vi "Fetch Repo Details.vi"(8 "error in (no error)":errorcluster) -> (0 "error out":errorcluster, 3 "Repo":refnum<class "Repo.lvclass">)   [LabVIEW 2020, in "Packages.lvlib" / "GPM.lvlib"]
uses:
  GPM.lvlib
  Repo_class/Repo.lvclass
  Repo_class/RepoType--enum.ctl
  Repo_class/Repo.lvclass/Repo.ctl
  Repo_class/Write Name.vi
  Repo_class/Write RepoType.vi
  Repo_class/Write URL.vi
  Repo_class/Write LastUpdated.vi
  <vilib>/addons/database/Connection.llb/DB Tools Open Connec (String).vi
  <vilib>/addons/database/_DB Variant To Data/Database Variant To Data.xnode
  <vilib>/addons/database/NI_Database_API.lvlib
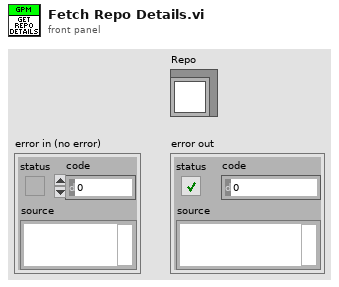
[diagram p1: front panel]
types:
  T1 = typedef "Packages.lvlib/Repo.lvclass/RepoType--enum.ctl" = enum16{"VIPM", "NIPM", "GPM"}
  T2 = typedef "NI_Database_API.lvlib/Conn ObjectReference.ctl" = refnum<k1>
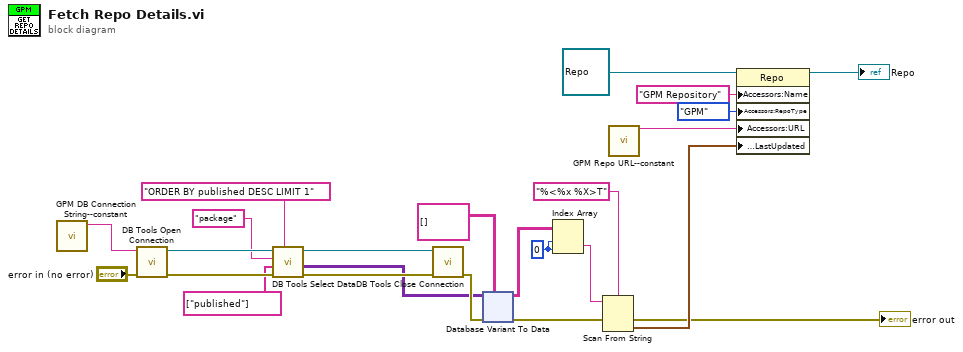
[diagram p0: block diagram]
diagram:
  w12 = 0 ("disabled index (col)")
  n1 = call "GPM DB Connection String--constant.vi"() -> ("DB Connection String"=w5:string)  [unwired: 11 in]
  n2 = call-poly <vilib>:"DB Tools Open Connection.vi"("error in (no error)"="error in (no error)", "connection information"=w5) -> ("error out"=w24:errorcluster, "connection reference"=w14:T2)  [unwired: 6 in]
  n3 = call <vilib>:"DB Tools Select Data.vi"("condition"="ORDER BY published DESC LIMIT 1", "error in (no error)"=w24, "columns"=string[] ["published"], "table"="package", "connection reference"=w14) -> ("error out"=w22:errorcluster, "data"=w20:variant[][], "connection reference out"=w23:T2)  [unwired: 1 in]
  n4 = call <vilib>:"DB Tools Close Connection.vi"("error in (no error)"=w22, "connection reference"=w23) -> ("error out"=w21:errorcluster)  [unwired: 5 in]
  n5 = xnode "Database Variant To Data"("database variant"=w20, "error in (no error)"=w21, "type"=string[][] []) -> ("data"=w17:string[][], "error out"=w11:errorcluster)
  n6 = Index Array(array=w17, index (row)=w12, index (col)=w12) -> (element=w10:string)
  n7 = Scan From String(format string="%<%x %X>T", input string=w10, error in=w11) -> (error out=→"error out":errorcluster, output 1=w3:timestamp)  [unwired: 2 in, 2 out]
  n8 = call "GPM Repo URL--constant.vi"() -> ("GPM Repo URL"=w4:string)  [unwired: 11 in]
  n9 = property class="Repo"(reference=refnum<class "Repo.lvclass"> refnum ("Repo in"), "Accessors:Name"="GPM Repository" ("Name"), "Accessors:RepoType"=RepoType--enum."GPM" ("RepoType"), "Accessors:URL"=w4, "Accessors:LastUpdated"=w3) -> (reference out=→"Repo":refnum<class "Repo.lvclass">)  [unwired: 1 in, 1 out]
